vi "Get Argument Info From Front Term.vi"(11 "Terminal in":refnum<vi>) -> (3 "Array":T1[](array[typedef]))   [LabVIEW 2017, in "CSM-Helper.lvclass"]
doc: "### Get Argument Info From Front Term.vi\n\n-- <b>Controls</b> --\n- <b>Terminal in</b>:\n\n-- <b>Indicators</b> --\n- <b>Array</b>:"
uses:
  CSM-Helper.lvclass
  Typedef/Def-Argument Info.ctl
  Utility/_Support/Terminals.llb/csmHelper-Terminals.lvlib
  _Shared/CSM Shared.lvlib
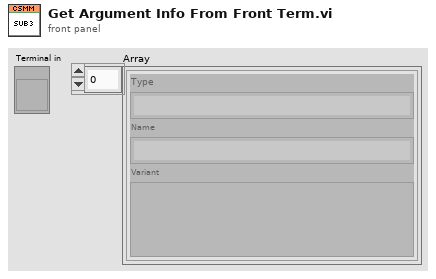
[diagram p1: front panel]
types:
  T1 = typedef "CSM-Helper.lvclass/Def-Argument Info.ctl" = cluster{"Type":string, "Name":string, "Variant":variant}
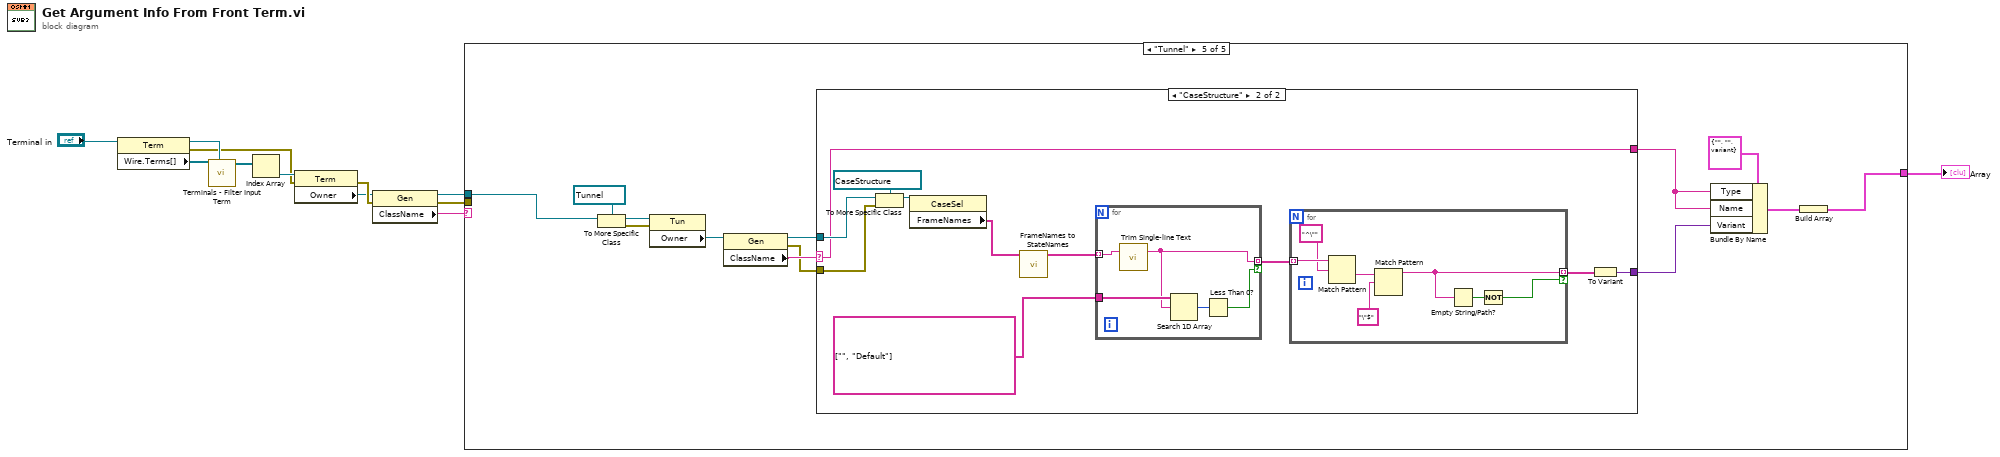
[diagram p0: block diagram]
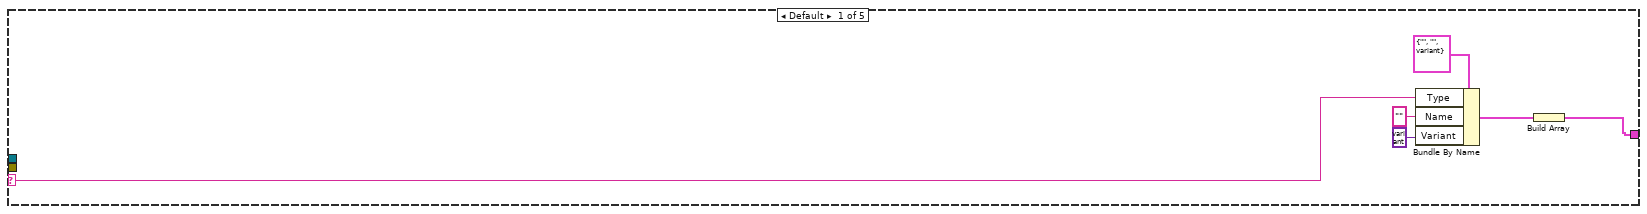
[diagram p2: hidden frame]
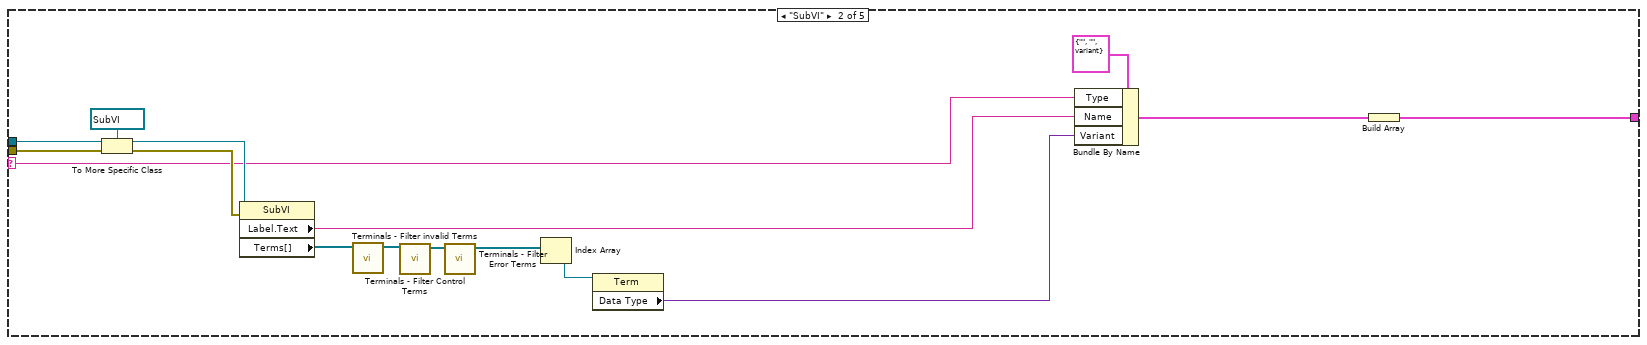
[diagram p3: hidden frame]
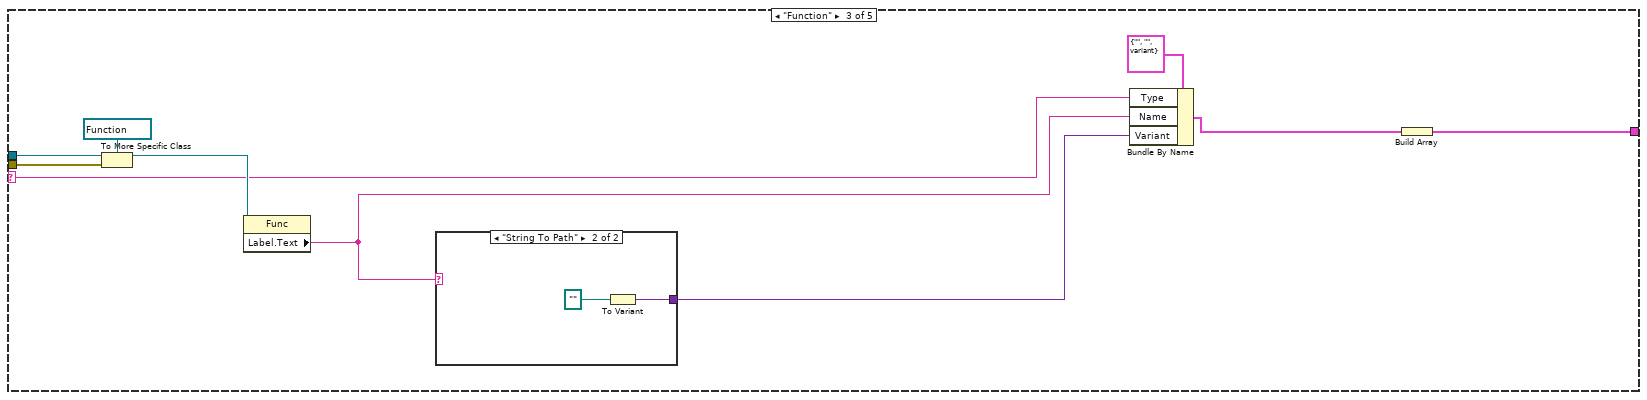
[diagram p4: hidden frame]
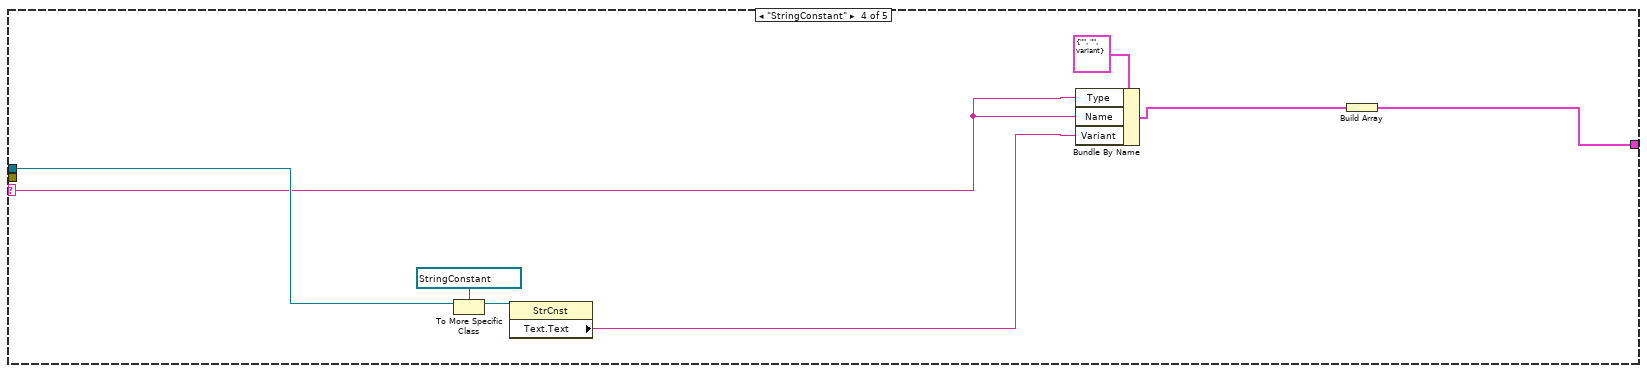
[diagram p6: hidden frame]
diagram:
  n1 = property class="Term"(reference="Terminal in") -> (reference out=w5:refnum<vi>, error out=w2:errorcluster, "Wire.Terms[]"=w6:refnum<vi>[])  [unwired: 1 in]
  n2 = call "Terminals - Filter Input Term.vi"("InnerTerminal in"=w5, "Wire.Terms[] in"=w6) -> ("Wire.Terms[] out"=w7:refnum<vi>[])  [unwired: 9 in]
  n3 = Index Array(array=w7) -> (element=w3:refnum<vi>)  [unwired: 1 in]
  n4 = property class="Term"(reference=w3, error in=w2) -> (error out=w11:errorcluster, "Owner"=w9:refnum<vi>)  [unwired: 1 out]
  n5 = property class="Gen"(reference=w9, error in=w11) -> (reference out=w10:refnum<vi>, error out=w8:errorcluster, "ClassName"=w12:string)
  n6 = case shown="\"Tunnel\"" w12 {
    selector: w12 -> [w18 w23 w39 w50 _]
    tunnel: w10 -> [_ w32 w42 w52 w67]
    tunnel: w8 -> [_ w31 w41 _ _]
    tunnel: [w13 w19 w35 w47 w55] -> w1
    frame Default {
      n7 = Bundle By Name(cluster=T1 {"Type"="", "Name"="", "Variant"=variant} ("Argument"), "Type"=w18, "Name"="", "Variant"=variant) -> (w15:T1)
      n8 = Build Array(w15) -> (w13:T1[])
    }
    frame "SubVI" {
      n9 = To More Specific Class(target class=refnum<vi> refnum ("reference out"), reference=w32, error in=w31) -> (specific class reference=w33:refnum<vi>, error out=w25:errorcluster)
      n10 = property class="SubVI"(reference=w33, error in=w25) -> ("Label.Text"=w22:string, "Terms[]"=w28:refnum<vi>[])  [unwired: 2 out]
      n11 = call "Terminals - Filter invalid Terms.vi"("Terms[]"=w28) -> ("Terms[] out"=w29:refnum<vi>[])  [unwired: 10 in]
      n12 = call "Terminals - Filter Control Terms.vi"("Terms[]"=w29) -> ("Terms[] out"=w30:refnum<vi>[])  [unwired: 10 in]
      n13 = call "Terminals - Filter Error Terms.vi"("Terms[]"=w30) -> ("Terms[] out"=w27:refnum<vi>[])  [unwired: 10 in]
      n14 = Index Array(array=w27) -> (element=w26:refnum<vi>)  [unwired: 1 in]
      n15 = property class="Term"(reference=w26) -> ("Data Type"=w21:variant)  [unwired: 1 in, 2 out]
      n16 = Bundle By Name(cluster=T1 {"Type"="", "Name"="", "Variant"=variant} ("Argument"), "Type"=w23, "Name"=w22, "Variant"=w21) -> (w20:T1)
      n17 = Build Array(w20) -> (w19:T1[])
    }
    frame "Function" {
      n18 = To More Specific Class(target class=refnum<vi> refnum ("reference out"), reference=w42, error in=w41) -> (specific class reference=w43:refnum<vi>)  [unwired: 1 out]
      n19 = property class="Func"(reference=w43) -> ("Label.Text"=w38:string)  [unwired: 1 in, 2 out]
      n20 = case shown="\"String To Path\"" w38 {
        tunnel: [_ w45] -> w37
        frame "False", Default {
        }
        frame "String To Path" {
          n21 = To Variant(anything=path "") -> (Variant=w45:variant)
        }
      }
      n22 = Bundle By Name(cluster=T1 {"Type"="", "Name"="", "Variant"=variant} ("Argument"), "Type"=w39, "Name"=w38, "Variant"=w37) -> (w36:T1)
      n23 = Build Array(w36) -> (w35:T1[])
    }
    frame "StringConstant" {
      n24 = To More Specific Class(target class=refnum<vi> refnum ("reference out"), reference=w52) -> (specific class reference=w54:refnum<vi>)  [unwired: 1 in, 1 out]
      n25 = property class="StrCnst"(reference=w54) -> ("Text.Text"=w49:string)  [unwired: 1 in, 2 out]
      n26 = Bundle By Name(cluster=T1 {"Type"="", "Name"="", "Variant"=variant} ("Argument"), "Type"=w50, "Name"=w50, "Variant"=w49) -> (w48:T1)
      n27 = Build Array(w48) -> (w47:T1[])
    }
    frame "Tunnel" {
      n28 = To More Specific Class(target class=refnum<vi> refnum ("reference out"), reference=w67) -> (specific class reference=w65:refnum<vi>, error out=w64:errorcluster)  [unwired: 1 in]
      n29 = property class="Tun"(reference=w65, error in=w64) -> ("Owner"=w63:refnum<vi>)  [unwired: 2 out]
      n30 = property class="Gen"(reference=w63) -> (reference out=w61:refnum<vi>, error out=w60:errorcluster, "ClassName"=w62:string)  [unwired: 1 in]
      n31 = case shown="\"CaseStructure\"" w62 {
        selector: w62 -> [w68 w74]
        tunnel: [_ w77] -> w57
        tunnel: w61 -> [_ w76]
        tunnel: w60 -> [_ w75]
        tunnel: [w68 w74] -> w58
        frame Default {
        }
        frame "CaseStructure" {
          n32 = To More Specific Class(target class=refnum<vi> refnum ("reference out"), reference=w76, error in=w75) -> (specific class reference=w79:refnum<vi>)  [unwired: 1 out]
          n33 = property class="CaseSel"(reference=w79) -> ("FrameNames"=w69:string[])  [unwired: 1 in, 2 out]
          n34 = call "FrameNames to StateNames.vi"("FrameNames"=w69) -> ("Array of Strings"=w70:string[])  [unwired: 10 in]
          n35 = for {
            tunnel: [w82] -> w71 mode=indexing if=w80
            tunnel: w70 -> [w84] mode=indexing
            tunnel: string[] ["", "Default"] ("items to filter") -> [w83]
            n36 = call "Trim Single-line Text.vi"("single-line text"=w84) -> ("trimed text"=w82:string)  [unwired: 2 in]
            n37 = Search 1D Array(1D array=w83, element=w82) -> (index of element=w81:i32)  [unwired: 1 in]
            n38 = Less Than 0?(x=w81) -> (x < 0?=w80:bool)
          }
          n39 = for {
            tunnel: w71 -> [w91] mode=indexing
            tunnel: [w87] -> w73 mode=indexing if=w86
            n40 = Match Pattern(string=w91, regular expression="^\"") -> (after substring=w89:string)  [unwired: 1 in, 3 out]
            n41 = Match Pattern(string=w89, regular expression="\"$") -> (before substring=w87:string)  [unwired: 1 in, 3 out]
            n42 = Empty String/Path?(string/path=w87) -> (empty?=w85:bool)
            n43 = Not(x=w85) -> (.not. x?=w86:bool)
          }
          n44 = To Variant(anything=w73) -> (Variant=w77:variant)
        }
      }
      n45 = Bundle By Name(cluster=T1 {"Type"="", "Name"="", "Variant"=variant} ("Argument"), "Type"=w58, "Name"=w58, "Variant"=w57) -> (w56:T1)
      n46 = Build Array(w56) -> (w55:T1[])
    }
  }
  "Array" <- w1
